vi "test1jj.vi"() -> ()   [LabVIEW 2018]
uses:
  <vilib>/imath/engines/lvmath2/RunTimeEngine/Managers/WorkSpace/UID Generator.vi
  <vilib>/imath/engines/lvmath2/RunTimeEngine/BuiltInFunctions/rand/NIMS_rand(1,I32).vi
  <vilib>/imath/engines/lvmath2/RunTimeEngine/RunTimeType/NIMS_RunTimeType_From StrictType (excl LVString).vi
  <instcachedir>/0/NIMS_RunTimeType_From StrictType (excl LVString)_E7E34A65C99947108168652BAD14964D.lvgen/NIMS_RunTimeType_From StrictType (excl LVString)_E7E34A65C99947108168652BAD14964D_000.vi
  <vilib>/imath/engines/lvmath2/RunTimeEngine/ErrorHandling/NIMS_Error From Error Code.vi
  <vilib>/imath/engines/lvmath2/RunTimeEngine/LocalVariableDefStatement/MC_LocalVariableDefStatement_Display.vi
  <vilib>/imath/engines/lvmath2/RunTimeEngine/BuiltInFunctions/density_kernel/NIMS_density_kernel(V,Var).vi
  <vilib>/imath/engines/lvmath2/RunTimeEngine/BuiltInFunctions/histogram/NIMS_[V]=histogram(V).vi
  <vilib>/imathl/engines/lvmath/Functions/Error Handling/Create Error.vi
  <vilib>/imath/engines/lvmath2/RunTimeEngine/IndexRead/NIMS M(S,$).vi
  <instcachedir>/0/NIMS M(S,$)_F24F360562DE41D8BE234322A2E15C65.lvgen/NIMS M(S,$)_F24F360562DE41D8BE234322A2E15C65_002.vi
  <instcachedir>/0/NIMS M(S,$)_F24F360562DE41D8BE234322A2E15C65.lvgen/NIMS M(S,$)_F24F360562DE41D8BE234322A2E15C65_000.vi
  <vilib>/imath/engines/lvmath2/RunTimeEngine/BuiltInFunctions/max/1 input/NIMS_max(RV).vi
  <instcachedir>/0/NIMS_max(RV)_237633DB1D604D5BA7001287DF3C7957.lvgen/NIMS_max(RV)_237633DB1D604D5BA7001287DF3C7957_000.vi
  <vilib>/imath/engines/lvmath2/RunTimeEngine/BuiltInFunctions/min/1 input/NIMS_min(RV).vi
  <instcachedir>/0/NIMS_min(RV)_EE2DD3E2888846108C5160A664B67832.lvgen/NIMS_min(RV)_EE2DD3E2888846108C5160A664B67832_000.vi
  <vilib>/imath/engines/lvmath2/RunTimeEngine/BuiltInFunctions/ones/NIMS_V=ones(I32,I32).vi
  <vilib>/imath/engines/lvmath2/RunTimeEngine/ArithmeticOperatorToken/NIMS_ArithmeticOperator_multmx(RV,CV).vi
  <instcachedir>/0/NIMS_ArithmeticOperator_multmx(RV,CV)_BD2DF24E790749FA8C1D6105F13E95CE.lvgen/NIMS_ArithmeticOperator_multmx(RV,CV)_BD2DF24E790749FA8C1D6105F13E95CE_000.vi
  <vilib>/imath/engines/lvmath2/RunTimeEngine/IndexReplace/NIMS V(S)=M.vi
  <instcachedir>/0/NIMS V(S)=M_E1EF42F6623D44DBA15317938B9EE7AF.lvgen/NIMS V(S)=M_E1EF42F6623D44DBA15317938B9EE7AF_001.vi
  <vilib>/imath/engines/lvmath2/RunTimeEngine/ErrorHandling/NIMS_Create Error From Enums.vi
  <vilib>/imath/engines/lvmath2/RunTimeEngine/ArithmeticOperatorToken/NIMS_ArithmeticOperator_times.vi
  <instcachedir>/0/NIMS_ArithmeticOperator_times_D7E4A7A4AD2C4409A0CE309D2741A5B4.lvgen/NIMS_ArithmeticOperator_times_D7E4A7A4AD2C4409A0CE309D2741A5B4_000.vi
  <vilib>/imath/engines/lvmath2/RunTimeEngine/Managers/SymbolTable/Clear UID.vi
  <vilib>/imath/engines/lvmath2/RunTimeEngine/NodeEndStatement/NIMS_NodeEndStatement_Output.vi
  <instcachedir>/0/NIMS_NodeEndStatement_Output_53EC0D466D134D7ABD903AC30B43404B.lvgen/NIMS_NodeEndStatement_Output_53EC0D466D134D7ABD903AC30B43404B_010.vi
  <instcachedir>/0/NIMS_NodeEndStatement_Output_53EC0D466D134D7ABD903AC30B43404B.lvgen/NIMS_NodeEndStatement_Output_53EC0D466D134D7ABD903AC30B43404B_005.vi
  <vilib>/imath/engines/lvmath2/RunTimeEngine/ErrorHandling/NIMS_Finalize Error.vi
  <vilib>/imath/engines/lvmath2/RunTimeEngine/Managers/SymbolTable/NIMS_WorkSpace.lvlib
panel:
  out "point":dbl[](graph)
  out "min":dbl
  out "max":dbl
  out "all":cluster{"t":dbl[], "y":dbl[]}[](graph)
  out "hist Gaussian":cluster{"BIN":dbl[], "N":dbl[]}(graph)
  out "Ideal gaussian":cluster{"xi":dbl[], "f":dbl[]}(graph)
  out "ksdensity Gaussian":cluster{"xi":dbl[], "f":dbl[]}(graph)
  out "line":dbl[](graph)
  out "m":dbl[](array[numeric])
  in  "num":dbl=10000.0
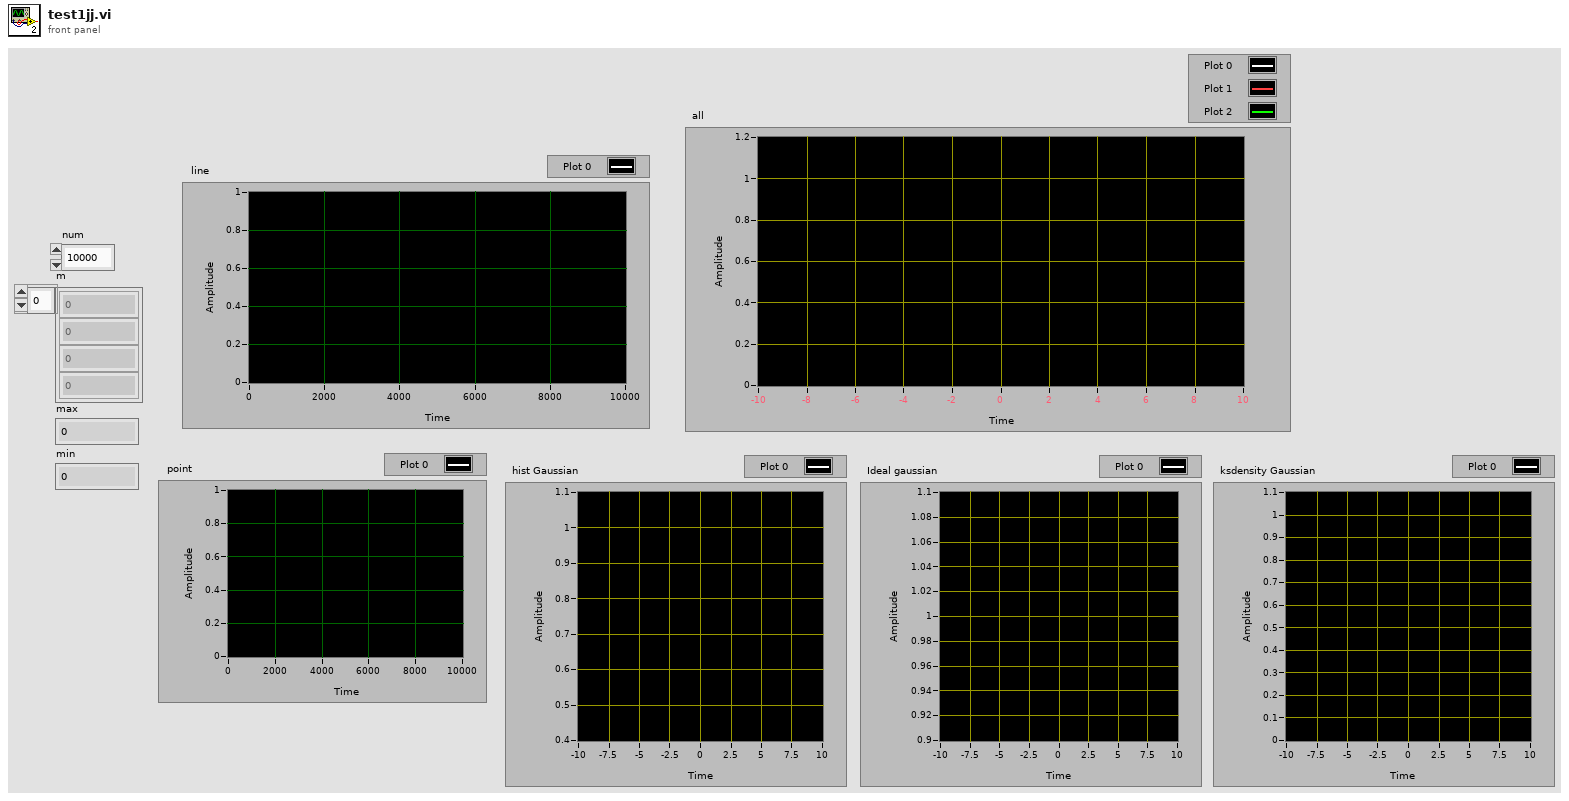
[diagram p1: front panel]
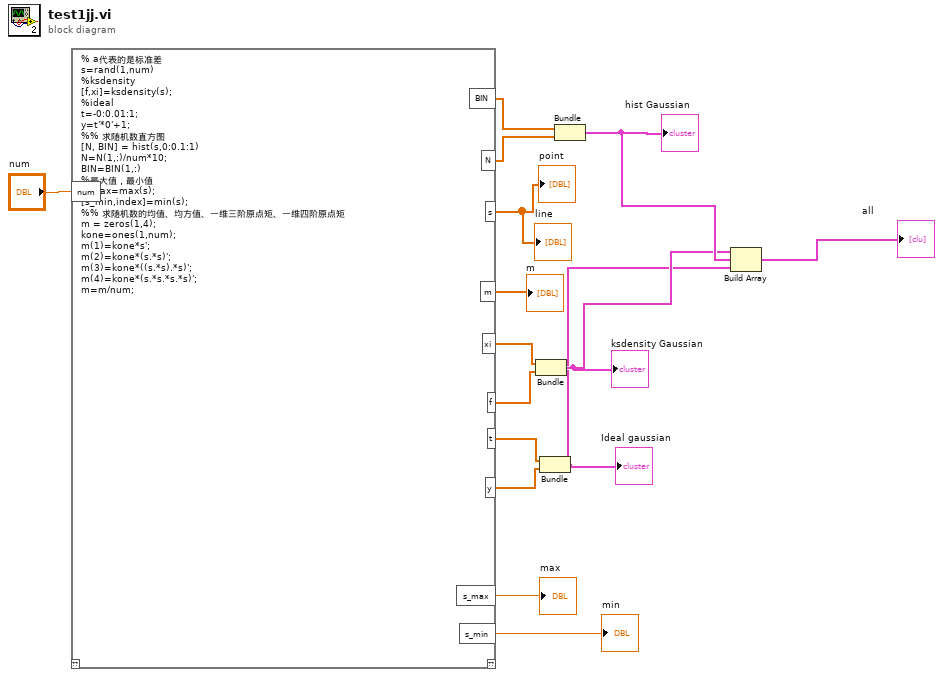
[diagram p0: block diagram]
diagram:
  n1 = mathscript code="% a代表的是标准差\ns=rand(1,num)\n%ksdensity\n[f,xi]=ksdensity(s);\n%ideal\nt=-0:0.01:1;\ny=t'*0'+1;\n%% 求随机数直方图\n[N, BIN] = hist(s,0:0.1:1)\nN=N(1,:)/num*10;\nBIN=BIN(1,:)\n%最大值，最小值\ns_max=max(s);\n[s_min,index]=min(s);\n%% 求随机数的均值、均方值、一维三阶原点矩、一维四阶原点矩\nm = zeros(1,4);        \nkone=ones(1,num);\nm(1)=kone*s';\nm(2)=kone*(s.*s)';\nm(3)=kone*((s.*s).*s)';\nm(4)=kone*(s.*s.*s.*s)';\nm=m/num;"("num"="num") -> ("m"=→"m":dbl[], "s"=→"line" →"point":dbl[], "xi"=w14:dbl[], "f"=w13:dbl[], "N"=w8:dbl[], "BIN"=w9:dbl[], "t"=w10:dbl[], "y"=w11:dbl[], "s_max"=→"max":sgl, "s_min"=→"min":sgl)  [unwired: 1 in, 1 out]
  n2 = Bundle("xi"=w14, "f"=w13) -> (w5:cluster{"xi":dbl[], "f":dbl[]})  [unwired: 1 in]
  "ksdensity Gaussian" <- w5
  n3 = Bundle("t"=w10, "y"=w11) -> (w4:cluster{"t":dbl[], "y":dbl[]})  [unwired: 1 in]
  "Ideal gaussian" <- w4
  n4 = Bundle("BIN"=w9, "N"=w8) -> (w6:cluster{"BIN":dbl[], "N":dbl[]})  [unwired: 1 in]
  "hist Gaussian" <- w6
  n5 = Build Array(w5, w6, w4) -> (→"all":cluster{"t":dbl[], "y":dbl[]}[])
